vi "Build Enumerations.vi"(7 "Enumerations in":map{string, T1}(c390), 8 "error in (no error)":errorcluster, 9 "Messages in":map{string, T5}(c390), 10 "Segments in":T3[](array[typedef]), 11 "ProtoParser in":refnum<class "ProtoParser.lvclass">) -> (0 "error out":errorcluster, 1 "Messages":map{string, T5}(c390), 2 "Segments":T3[](array[typedef]), 3 "ProtoParser out":refnum<class "ProtoParser.lvclass">, 5 "Enumerations":map{string, T1}(c390))   [LabVIEW 2020, in "LV-Protoc.lvlib" / "ProtoParser.lvclass"]
uses:
  ProtoParser.lvclass
  Raw Segment.ctl
  Segment Type.ctl
  LV-Proto/Message.ctl
  LV-Proto/Field.ctl
  LV-Proto/Type.ctl
  LV-Proto/Proto Type.ctl
  LV-Proto/Enumeration.ctl
  LV-Proto/Enum Value.ctl
  LV-Protoc.lvlib
  LV-Proto/LV-Proto.lvlib
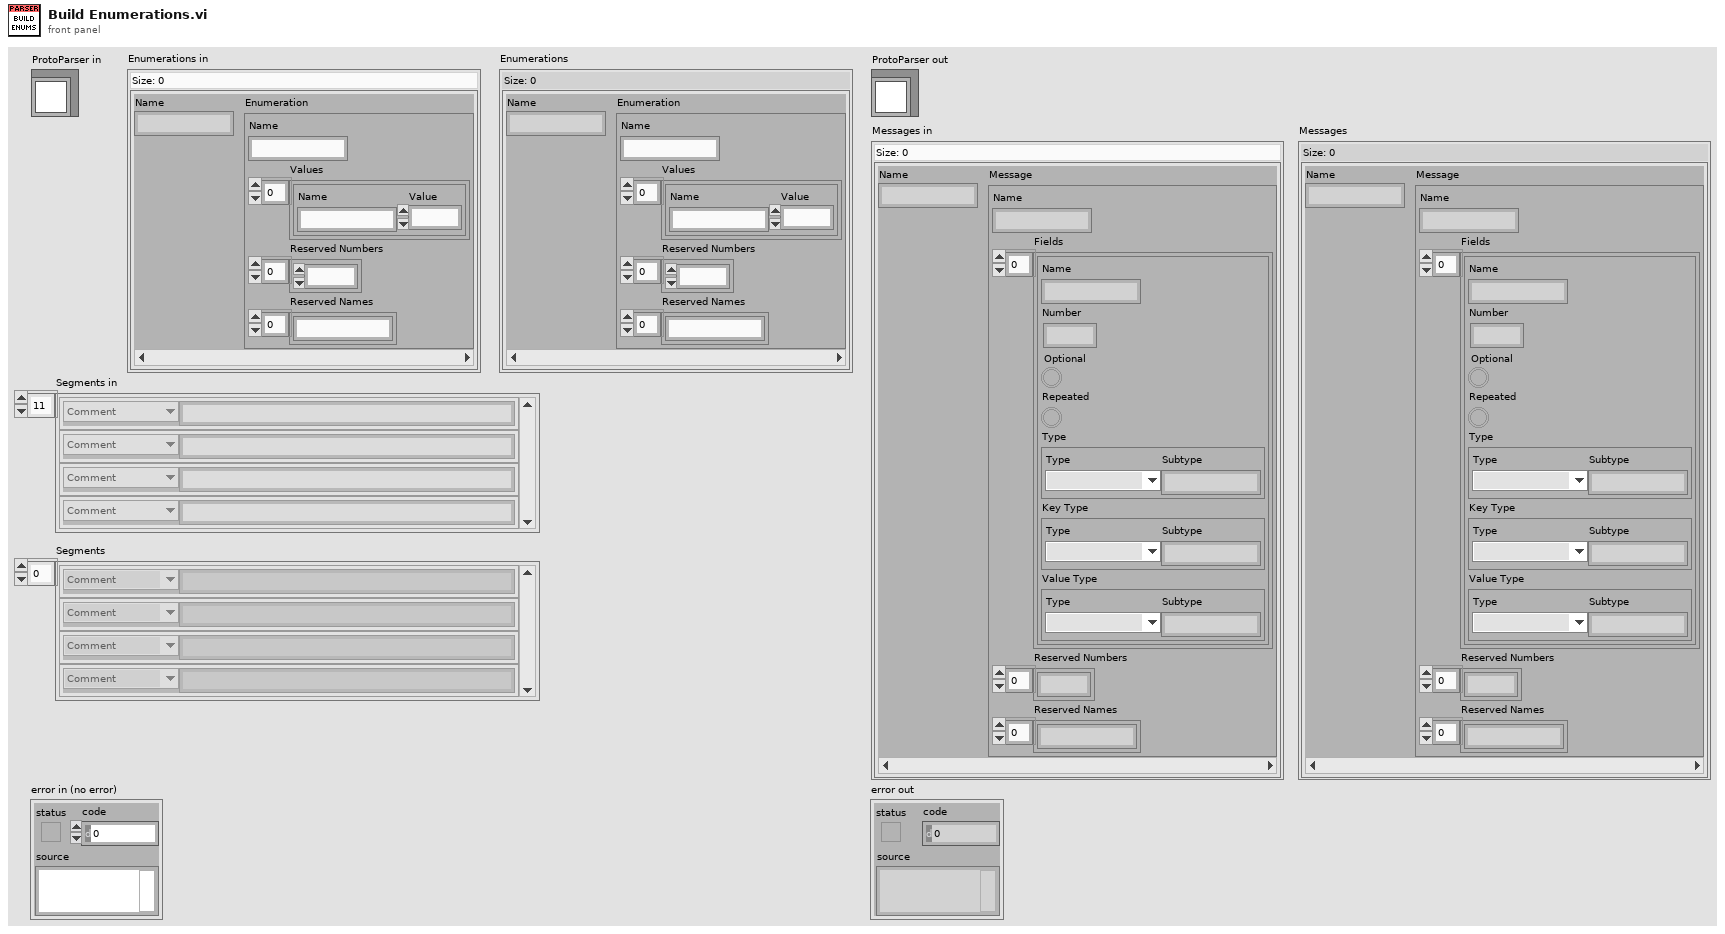
[diagram p1: front panel]
types:
  T1 = typedef "LV-Proto.lvlib/Enumeration.ctl" = cluster{"Name":string, "Values":T2[], "Reserved Numbers":u32[], "Reserved Names":string[]}
  T2 = typedef "LV-Proto.lvlib/Enum Value.ctl" = cluster{"Name":string, "Value":i32}
  T3 = typedef "LV-Protoc.lvlib/Raw Segment.ctl" = cluster{"Type":T4, "Text":string}
  T4 = typedef "LV-Protoc.lvlib/Segment Type.ctl" = enum16{"Comment", "Message Open", "Enum Open", "Message Close", "Enum Close", "Field", "Syntax", "Import", "Enum Value", "Package", "Reserved"}
  T5 = typedef "LV-Proto.lvlib/Message.ctl" = cluster{"Name":string, "Fields":T6[], "Reserved Numbers":u32[], "Reserved Names":string[]}
  T6 = typedef "LV-Proto.lvlib/Field.ctl" = cluster{"Name":string, "Number":u32, "Optional":bool, "Repeated":bool, "Type":T7, "Key Type":T7, "Value Type":T7}
  T7 = typedef "LV-Proto.lvlib/Type.ctl" = cluster{"Type":T8, "Subtype":string}
  T8 = typedef "LV-Proto.lvlib/Proto Type.ctl" = enum16{"UNKNOWN", "double", "float", "int32", "int64", "uint32", "uint64", "sint32", "sint64", "fixed32", "fixed64", "sfixed32", "sfixed64", "bool", "string", "bytes", "enum", "map", "message"}
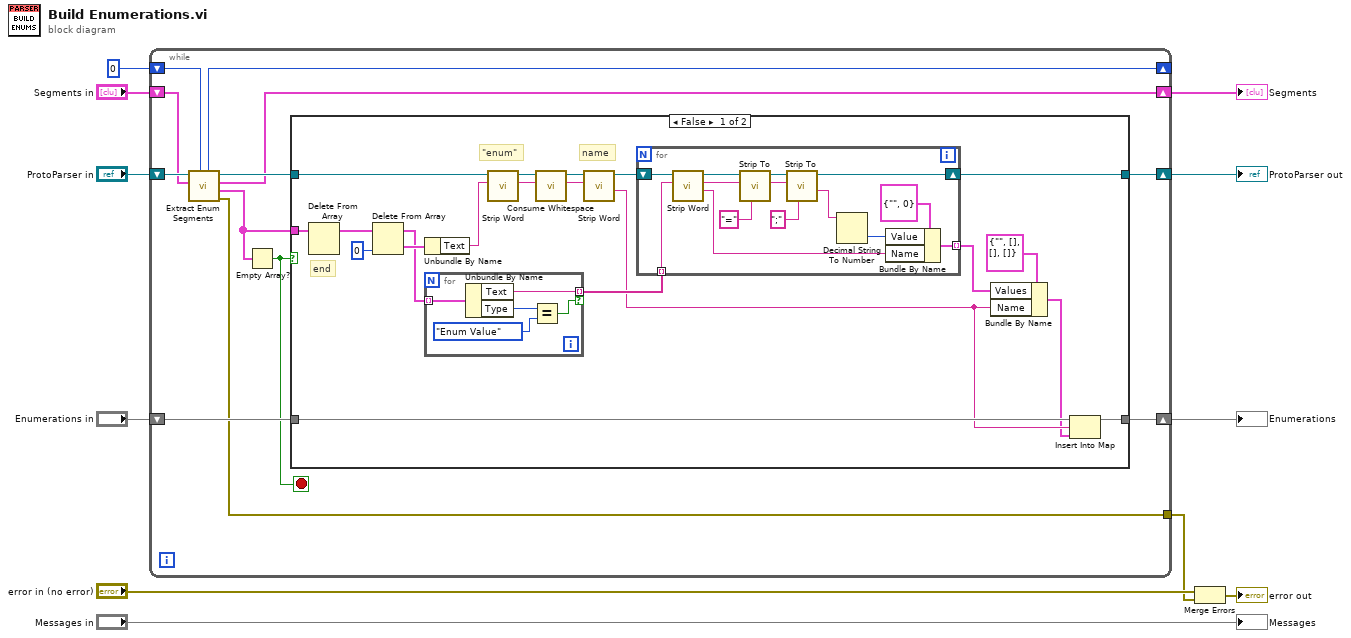
[diagram p0: block diagram]
diagram:
  n1 = while {
    shift-right: [w14] -> w9
    shift-left: "Segments in" -> [w22]
    shift-right: [w16] -> w7
    shift-left: "Enumerations in" -> [w17]
    shift-right: [w18] -> w5
    shift-left: "ProtoParser in" -> [w23]
    shift-right: [w19] -> _
    shift-left: 0 -> [w20]
    tunnel: [w13] -> w2
    stop <- w12 stop-if-true
    n2 = call "Extract Enum Segments.vi"("Start Index"=w20, "Segments in"=w22, "ProtoParser in"=w23) -> ("error out"=w13:errorcluster, "Enumeration Segments"=w15:T3[], "Remaining"=w14:T3[], "ProtoParser out"=w21:refnum<class "ProtoParser.lvclass">, "Next Index"=w19:i32)  [unwired: 4 in]
    n3 = Empty Array?(array=w15) -> (empty?=w12:bool)
    n4 = case shown="False" w12 {
      tunnel: w21 -> [w40 w63]
      tunnel: [w35 w63] -> w18
      tunnel: w17 -> [w33 w64]
      tunnel: [w32 w64] -> w16
      tunnel: w15 -> [w29 _]
      frame False {
        # "end"
        # "name"
        # "\"enum\""
        n5 = Delete From Array(array=w29) -> (array with subset deleted=w43:T3[])  [unwired: 2 in, 1 out]
        n6 = Delete From Array(array=w43, index=0) -> (deleted portion=w41:T3, array with subset deleted=w38:T3[])  [unwired: 1 in]
        n7 = Unbundle By Name(w41) -> ("Text"=w39:string)
        n8 = for {
          tunnel: w38 -> [w62] mode=indexing
          tunnel: [w59] -> w37 mode=indexing if=w58
          n9 = Unbundle By Name(w62) -> ("Text"=w59:string, "Type"=w61:T4)
          n10 = Equal?(x=w61, y=Segment_Type."Enum Value") -> (x = y?=w58:bool)
        }
        n11 = call "Strip Word.vi"("String"=w39, "ProtoParser in"=w40) -> ("Remaining"=w26:string, "ProtoParser out"=w28:refnum<class "ProtoParser.lvclass">)  [unwired: 6 in, 2 out]
        n12 = call "Consume Whitespace.vi"("String"=w26, "ProtoParser in"=w28) -> ("Remaining"=w25:string, "ProtoParser out"=w27:refnum<class "ProtoParser.lvclass">)  [unwired: 7 in, 1 out]
        n13 = call "Strip Word.vi"("String"=w25, "ProtoParser in"=w27) -> ("Word"=w30:string, "ProtoParser out"=w36:refnum<class "ProtoParser.lvclass">)  [unwired: 6 in, 2 out]
        n14 = for {
          tunnel: w37 -> [w56] mode=indexing
          shift-right: [w46] -> w35
          shift-left: w36 -> [w57]
          tunnel: [w44] -> w34 mode=indexing
          n15 = call "Strip Word.vi"("String"=w56, "ProtoParser in"=w57) -> ("Word"=w45:string, "Remaining"=w54:string, "ProtoParser out"=w55:refnum<class "ProtoParser.lvclass">)  [unwired: 6 in, 1 out]
          n16 = call "Strip To.vi"("End"="=", "String"=w54, "ProtoParser in"=w55) -> ("Remaining"=w51:string, "ProtoParser out"=w52:refnum<class "ProtoParser.lvclass">)  [unwired: 5 in, 2 out]
          n17 = call "Strip To.vi"("End"=";", "String"=w51, "ProtoParser in"=w52) -> ("Portion"=w49:string, "ProtoParser out"=w46:refnum<class "ProtoParser.lvclass">)  [unwired: 5 in, 2 out]
          n18 = Decimal String To Number(string=w49) -> (number=w47:i32)  [unwired: 2 in, 1 out]
          n19 = Bundle By Name(cluster=T2 {"Name"="", "Value"=0} ("Enum Value"), "Value"=w47, "Name"=w45) -> (w44:T2)
        }
        n20 = Bundle By Name(cluster=T1 {"Name"="", "Values"=[], "Reserved Numbers"=[], "Reserved Names"=[]} ("Enumeration"), "Values"=w34, "Name"=w30) -> (w24:T1)
        n21 = Insert Into Map(map in=w33, key=w30, value=w24) -> (map out=w32:map{string, T1})  [unwired: 2 out]
      }
      frame True {
      }
    }
  }
  "ProtoParser out" <- w5
  "Segments" <- w9
  "Enumerations" <- w7
  n22 = Merge Errors("error in (no error)", w2) -> (→"error out":errorcluster)
  "Messages" <- "Messages in"
